vi "Write Idioma.vi"(8 "error in (no error)":errorcluster, 10 "Idioma":enum16{"Español", "Ingles"}(ring), 11 "Cafe in":refnum<class "Cafe.lvclass">) -> (0 "error out":errorcluster, 3 "Cafe out":refnum<class "Cafe.lvclass">)   [LabVIEW 2020, in "Cafe.lvlib" / "Cafe.lvclass"]
uses:
  Cafe.lvclass
  Cafe.lvclass/Cafe.ctl
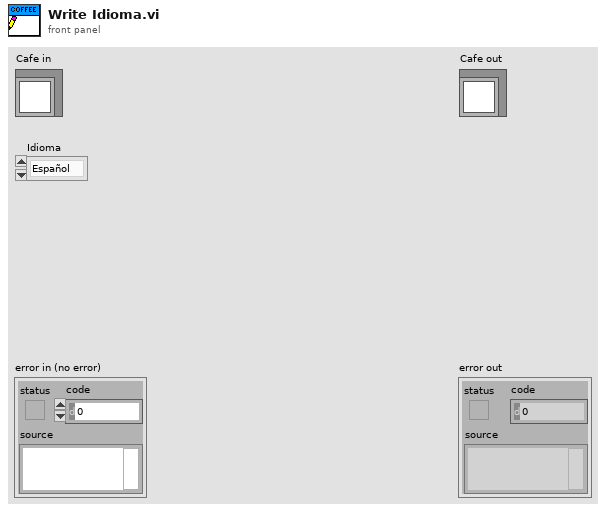
[diagram p1: front panel]
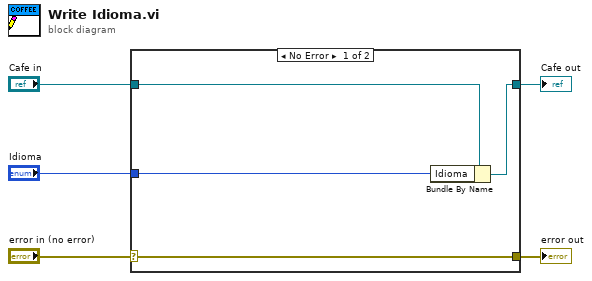
[diagram p0: block diagram]
diagram:
  n1 = case shown="No Error" "error in (no error)" {
    selector: "error in (no error)" -> [w9 w10]
    tunnel: [w9 w10] -> w4
    tunnel: [w7 w11] -> w2
    tunnel: "Cafe in" -> [w8 w11]
    tunnel: "Idioma" -> [w6 _]
    frame No Error {
      n2 = Bundle By Name(cluster=w8, "Idioma"=w6) -> (w7:refnum<class "Cafe.lvclass">)
    }
    frame Error {
    }
  }
  "error out" <- w4
  "Cafe out" <- w2
